vi "hiz_denetim_sistemi.vi"() -> ()   [LabVIEW 2020]
uses:
  <vilib>/Instr/_visa.llb/VISA Configure Serial Port (Instr).vi
  <vilib>/smtpClient/Set Message Text.vi
  <vilib>/smtpClient/LabVIEWSMTPClient.lvlib
panel:
  in  "tAlıcı (mail)o":string[](array[string])
  in  "Şifre":string
  in  "Gönderen (mail)":string
  out "TARİH & SAAT":timestamp
  out "String":string
  in  "UYGULAMA\nSONLANDIR":bool
  in  "VISA resource name":refnum<visa-resource-name>
  # "T.C KARAYOLLARI GENEL MÜDÜRLÜĞÜ\nKASTAMONU-AĞLI OTOYOLU \nELEKTRONİK HIZ DENETLEME SİSTEMİ KONTROL EKRANI"
  # "MAİL AYARLARI"
  # "AYARLAR"
  # "70"
  # "SERİ PORT SEÇİM"
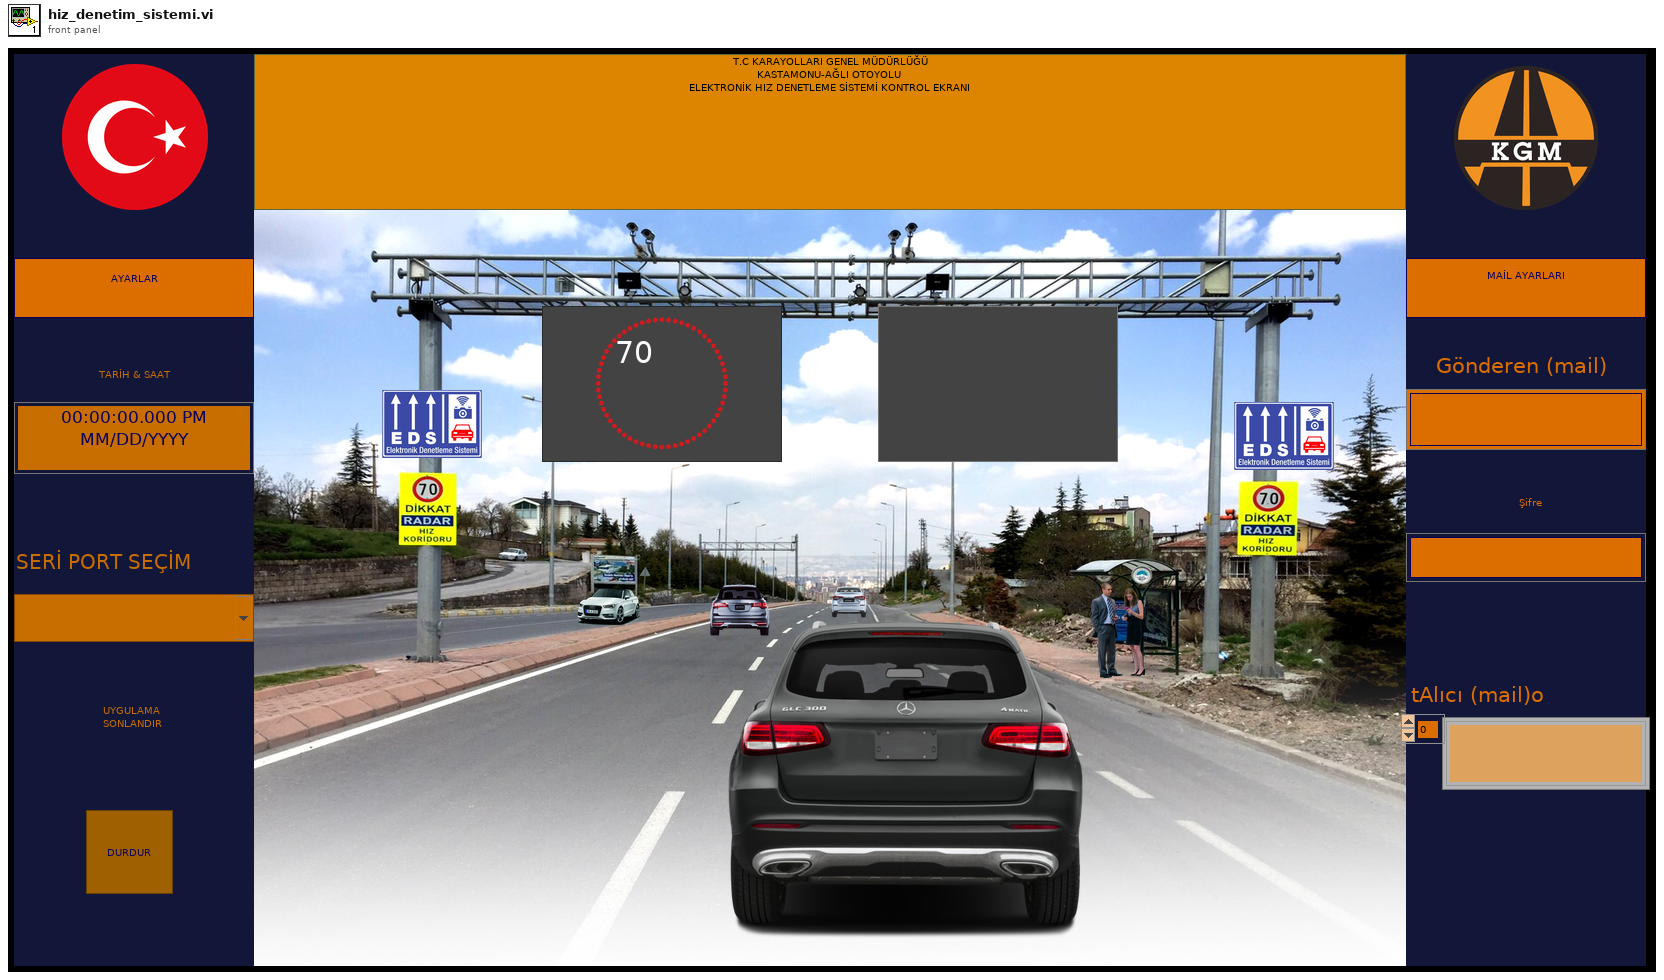
[diagram p1: front panel]
types:
  T1 = typedef "LabVIEWSMTPClient.lvlib/SmtpClientHandle.ctl" = refnum<k1>
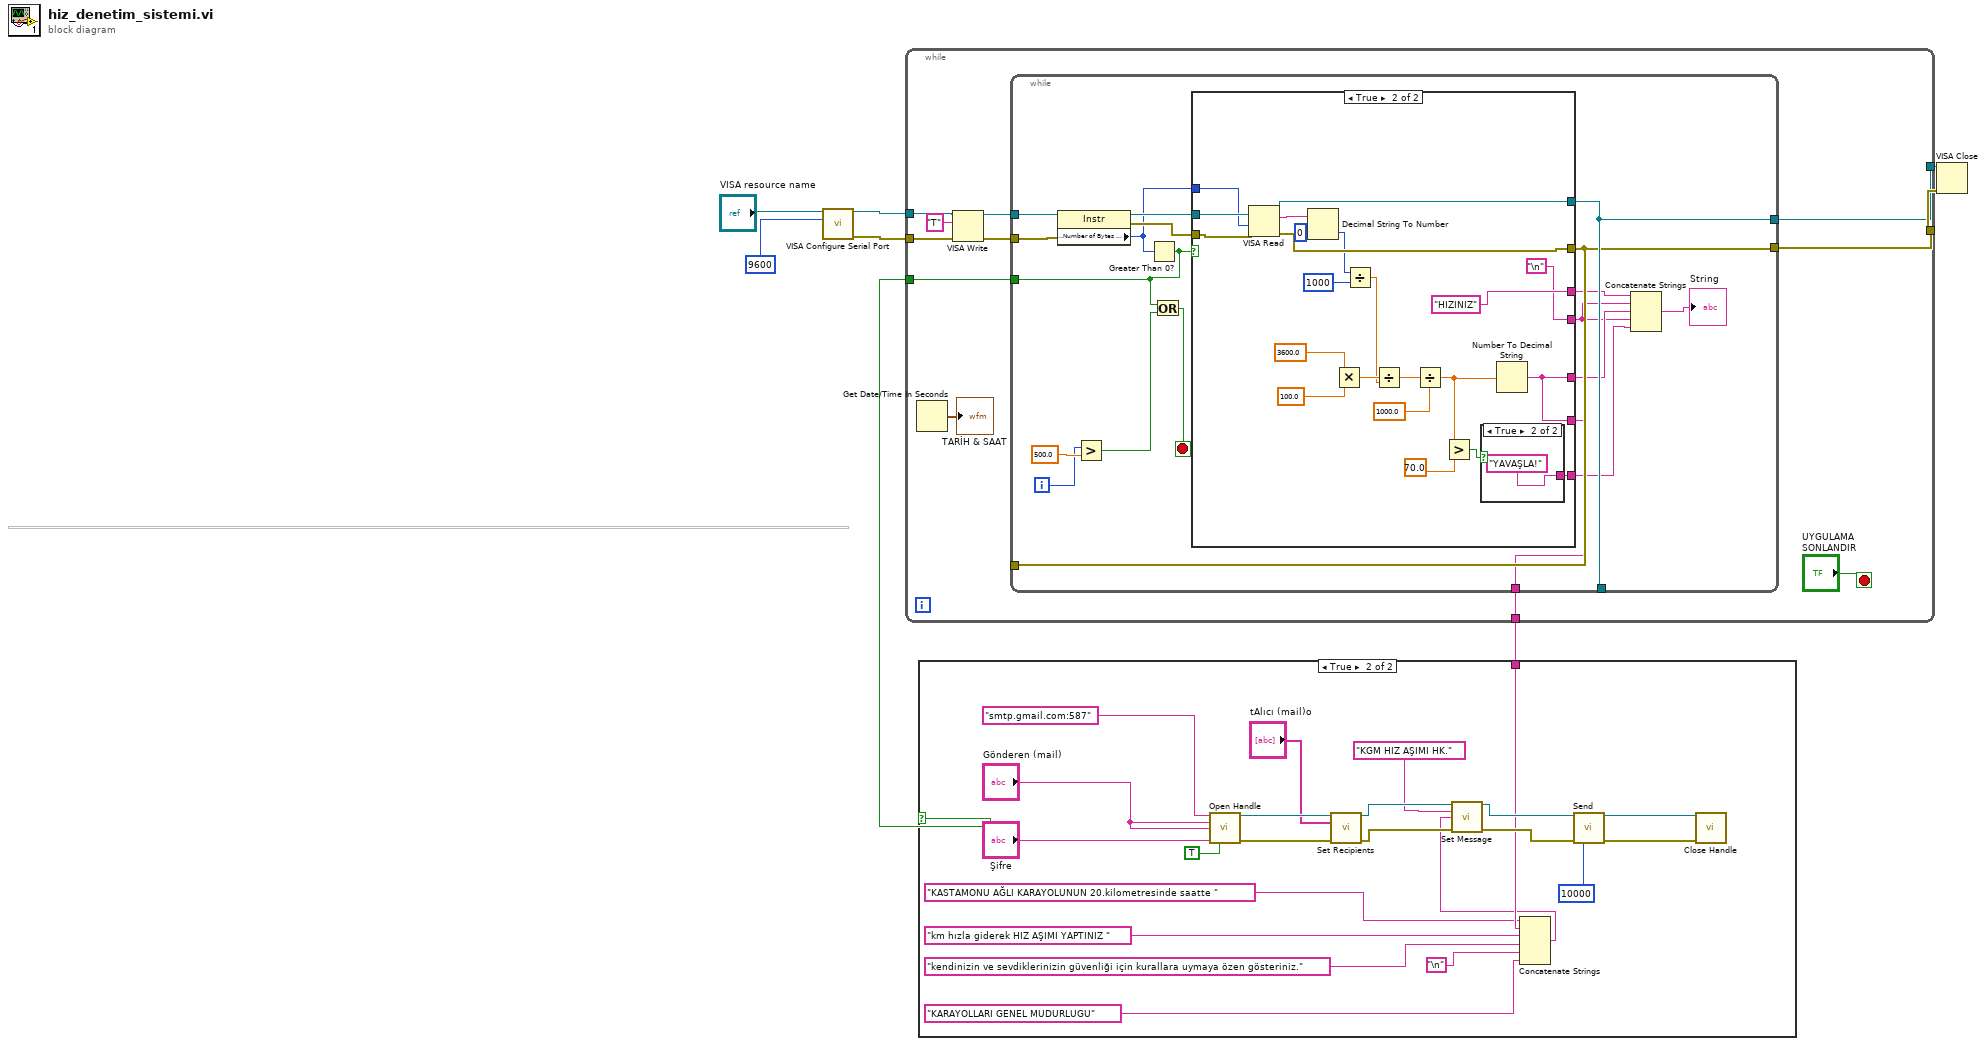
[diagram p0: block diagram]
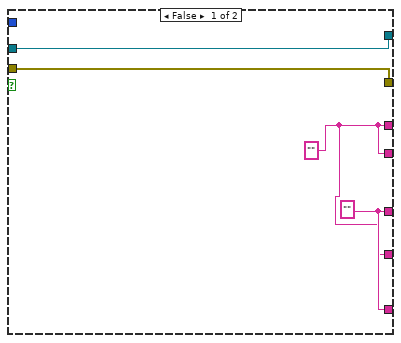
[diagram p3: hidden frame]
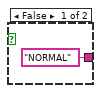
[diagram p4: hidden frame]
diagram:
  n1 = call-poly "VISA Configure Serial Port"("VISA resource name"="VISA resource name", "baud rate (9600)"=u32 9600) -> ("VISA resource name out"=w6:refnum<visa-resource-name>, "error out"=w5:errorcluster)  [unwired: 12 in]
  n2 = while {
    tunnel: w6 -> [w19]
    tunnel: w5 -> [w18]
    tunnel: [w13] -> w4
    tunnel: [w12] -> w3
    tunnel: [w10] -> w2
    tunnel: [w9] -> w1
    stop <- "UYGULAMA\nSONLANDIR" stop-if-true
    n3 = Get Date/Time In Seconds() -> (seconds since 1Jan1904=→"TARİH & SAAT":timestamp)
    n4 = VISA Write(VISA resource name=w19, write buffer="T", error in (no error)=w18) -> (VISA resource name out=w16:refnum<visa-resource-name>, error out=w15:errorcluster)  [unwired: 1 out]
    n5 = while {
      tunnel: w16 -> [w37]
      tunnel: w15 -> [w36]
      tunnel: [w28] -> _
      tunnel: [w27] -> _
      tunnel: [w28] -> w13
      tunnel: [w27] -> w12
      tunnel: [w21] -> w10
      tunnel: [w20] -> w9
      i -> [w31]
      stop <- w29 stop-if-true
      n6 = property class="Instr"(reference=w37, error in=w36) -> (reference out=w35:refnum<visa-resource-name>, error out=w34:errorcluster, "Serial Settings:Number of Bytes at Serial Port"=w33:u32)
      n7 = Greater?(x=w31, y=500.0) -> (0:w30:bool)
      n8 = Greater Than 0?(x=w33) -> (x > 0?=w21:bool)
      n9 = Or(x=w21, y=w30) -> (x .or. y?=w29:bool)
      n10 = case shown="True" w21 {
        tunnel: w35 -> [w41 w62]
        tunnel: w34 -> [w40 w61]
        tunnel: w33 -> [_ w60]
        tunnel: [w41 w58] -> w28
        tunnel: [w40 w57] -> w27
        tunnel: [w38 "HIZINIZ" ("string")] -> w26
        tunnel: [w39 w42] -> w25
        tunnel: [w39 w44] -> w24
        tunnel: [w38 "\n"] -> w23
        tunnel: [w38 w42] -> w20
        frame False {
          w39 = "" ("string")
          w38 = "" ("string")
        }
        frame True {
          (unwired) 0 ("number")
          n11 = VISA Read(VISA resource name=w62, byte count=w60, error in (no error)=w61) -> (VISA resource name out=w58:refnum<visa-resource-name>, read buffer=w59:string, error out=w57:errorcluster)  [unwired: 1 out]
          n12 = Decimal String To Number(string=w59) -> (number=w56:i32)  [unwired: 2 in, 1 out]
          n13 = Multiply(x=3600.0 ("y"), y=100.0) -> (x*y=w50:dbl)
          n14 = Divide(x=w56, y=1000) -> (x/y=w49:dbl)
          n15 = Divide(x=w50, y=w49) -> (x/y=w54:dbl)
          n16 = Divide(x=w54, y=1000.0) -> (x/y=w47:dbl)
          n17 = Greater?(x=w47, y=70.0) -> (0:w45:bool)
          n18 = case shown="True" w45 {
            tunnel: ["NORMAL" ("string") "YAVAŞLA!" ("string")] -> w44
            frame False {
            }
            frame True {
            }
          }
          n19 = Number To Decimal String(number=w47) -> (decimal integer string=w42:string)  [unwired: 1 in]
        }
      }
      n20 = Concatenate Strings(w26, w23, w25, w23, w24) -> (→"String":string)
    }
  }
  n21 = case shown="True" w2 {
    tunnel: w1 -> [_ w73]
    frame False {
    }
    frame True {
      n22 = call <vilib>:"Open Handle.vi"("server address"="smtp.gmail.com:587", "from"="Gönderen (mail)", "username"="Gönderen (mail)", "password"="Şifre", "use TLS (false)"=TRUE) -> ("handle out"=w86:T1, "error out"=w82:errorcluster)  [unwired: 9 in]
      n23 = call <vilib>:"Set Recipients.vi"("handle in"=w86, "to"="tAlıcı (mail)o", "error in (no error)"=w82) -> ("handle out"=w85:T1, "error out"=w81:errorcluster)  [unwired: 11 in]
      n24 = Concatenate Strings("KASTAMONU AĞLI KARAYOLUNUN 20.kilometresinde saatte " ("plain text message"), w73, "km hızla giderek HIZ AŞIMI YAPTINIZ " ("plain text message"), "kendinizin ve sevdiklerinizin güvenliği için kurallara uymaya özen gösteriniz." ("plain text message"), "\n", "KARAYOLLARI GENEL MUDURLUGU" ("plain text message")) -> (w65:string)
      n25 = call-poly <vilib>:"Set Message.vi"("handle in"=w85, "subject"="KGM HIZ AŞIMI HK.", "plain text message"=w65, "error in (no error)"=w81) -> ("handle out"=w84:T1, "error out"=w80:errorcluster)  [unwired: 10 in]
      n26 = call <vilib>:"Send.vi"("handle in"=w84, "error in (no error)"=w80, "timeout in ms (10000)"=10000) -> ("handle out"=w83:T1, "error out"=w79:errorcluster)  [unwired: 10 in, 1 out]
      n27 = call <vilib>:"Close Handle.vi"("handle in"=w83, "error in (no error)"=w79) -> ()  [unwired: 12 in, 2 out]
    }
  }
  n28 = VISA Close(VISA resource name=w4, error in (no error)=w3) -> ()  [unwired: 1 out]
